vi "总磷氨氮测量数据储存.vi"   [LabVIEW 2016, in "氨氮.lvlib"]
types:
  T1 = cluster{"时间标识":timestamp, "监测值":sgl, "单位":u16, "数据标识":string, "因子编码":u32, "标样参考值":sgl, "F0":sgl, "F1":sgl, "F2":sgl, "F3":sgl, "温度":sgl, "湿度":sgl, "量程标识":string}
  T2 = enum16{"维护数据", "水样测试", "标样核查", "零点核查", "跨度核查", "空白测试", "平行样测试", "加标回收", "空白校准", "标样校准", "初始化（清洗）"}
  T3 = cluster{"系统时间":timestamp, "工作状态":enum16{"空闲", "水样测试", "标样核查", "零点核查", "跨度核查", "空白测试", "平行样测试", "加标回收", "空白校准", "标样校准", "初始化（清洗）"}, "测量模式":enum16{"待机", "连续模式", "周期模式", "定点模式", "受控模式", "手动模式"}, "告警代码":enum16{"无告警", "缺试剂告警", "缺水样告警", "缺蒸馏水告警", "缺标液告警", "仪表漏液告警", "标定异常告警", "超量程告警", "加热异常", "低试剂预警", "超上限告警", "超下限告警", "仪表内部其他异常", "滴定异常告警", "电极异常告警", "量程切换告警", "参数设置告警", "PH电极电位异常", "电导率电极异常", "浊度光度异常", "溶解氧电极异常", "溶解氧光强异常", "温度异常告警", "PH异常告警", "溶解氧异常告警", "电导率异常告警", "浊度异常告警", "叶绿素异常告警", "藻密度异常告警", "蓝绿藻异常告警", "ORP异常告警", "氨氮异常告警", "清洁刷异常告警", "SD卡异常告警", "蓝牙异常告警", "Wifi异常告警", "流程异常告警"}, "故障代码":enum16{"无故障", "电机故障", "温度故障", "通讯故障", "滴定故障"}, "日志代码":u16, "软件版本":u16, "F0":sgl, "F1":sgl, "F2":sgl, "F3":sgl, "T":sgl, "H":sgl, "id":u16, "flowid":u16, "量程":u16, "总磷控温温度1":sgl, "营养盐控温温度2":sgl, "ADC":sgl}
  T4 = enum16{"空闲", "水样测试", "标样核查", "零点核查", "跨度核查", "空白测试", "平行样测试", "加标回收", "空白校准", "标样校准", "初始化（清洗）"}
  T5 = cluster{"跨度值":dbl, "零点标准液浓度":dbl, "跨度标准液浓度":dbl, "标准液标准浓度":dbl}
  T6 = cluster{"因子编码":u32, "单位":u16, "标样参考值":sgl, "水样数据时间":timestamp, "水样实测值":sgl, "水样数据标识":string, "标样数据时间":timestamp, "标样实测值":sgl, "标样数据标识":string, "空白数据时间":timestamp, "空白实测值":sgl, "空白数据标识":string, "零点核查数据时间":timestamp, "零点核查实测值":sgl, "零点核查数据标识":string, "跨度核查数据时间":timestamp, "跨度核查实测值":sgl, "跨度核查数据标识":string, "加标回收数据时间":timestamp, "加标回收实测值":sgl, "加标回收数据标识":string, "平行样数据时间":timestamp, "平行样实测值":sgl, "平行样数据标识":string}
  T7 = cluster{"运行模式":enum16{"维护模式", "常规模式", "应急模式", "质控模式"}}
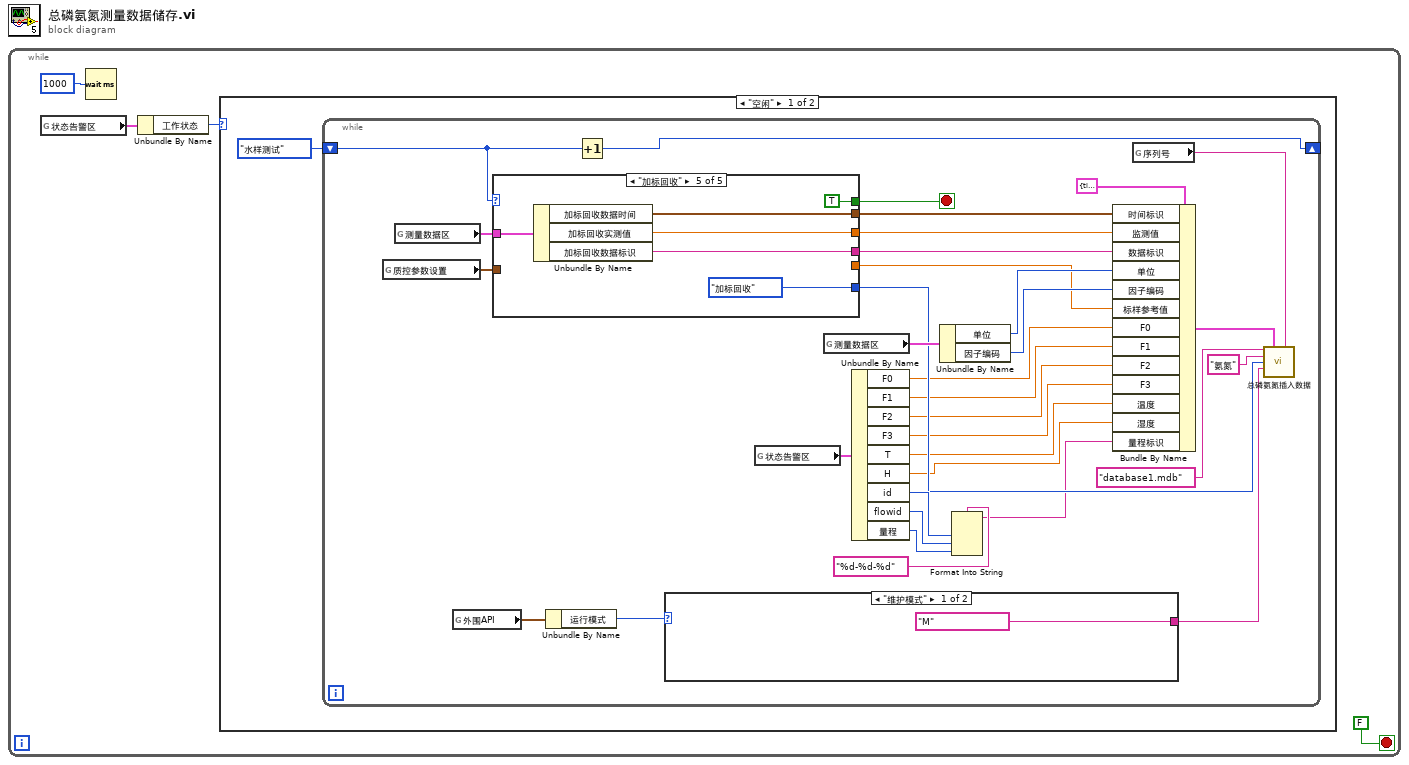
[diagram p0: block diagram]
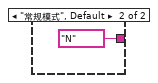
[diagram p2: hidden frame]
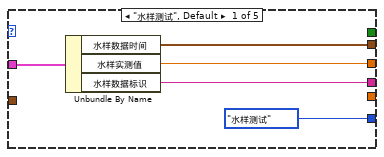
[diagram p3: hidden frame]
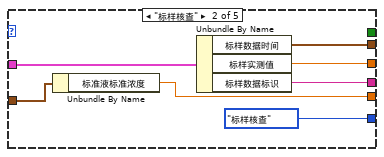
[diagram p4: hidden frame]
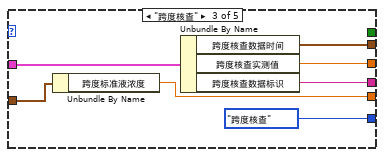
[diagram p5: hidden frame]
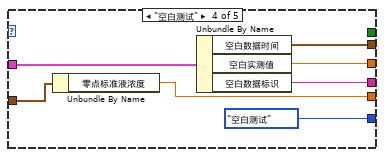
[diagram p6: hidden frame]
diagram:
  n1 = while {
    stop <- FALSE stop-if-true
    n2 = global read "VAR氨氮全局变量.vi" "状态告警区"() -> (w3:T3)
    n3 = Wait (ms)(milliseconds to wait=u32 1000 ("等待时间（毫秒）")) -> ()  [unwired: 1 out]
    n4 = Unbundle By Name(w3) -> ("工作状态"=w2:T4)
    n5 = case shown="\"空闲\"" w2 {
      frame "空闲" {
        n6 = while {
          shift-right: [w32] -> _
          shift-left: enum16{"水样测试", "标样核查", "跨度核查", "空白测试", "加标回收"}."水样测试" ("测量模式") -> [w33]
          stop <- w34 stop-if-true
          n7 = global read "氨氮断电保存全局变量.vi" "质控参数设置"() -> (w7:T5)
          n8 = global read "VAR氨氮全局变量.vi" "测量数据区"() -> (w26:T6)
          n9 = global read "VAR氨氮全局变量.vi" "外围API"() -> (w10:T7)
          n10 = case shown="\"加标回收\"" w33 {
            tunnel: w26 -> [w41 w48 w55 w62 w67]
            tunnel: [w45 w52 w59 w66 w72] -> w31
            tunnel: [w44 w51 w58 w65 w71] -> w30
            tunnel: [w43 w50 w57 w64 w70] -> w29
            tunnel: [T2."水样测试" ("测量模式") T2."标样核查" ("测量模式") T2."跨度核查" ("测量模式") T2."空白测试" ("测量模式") T2."加标回收" ("测量模式")] -> w18
            tunnel: [_ _ _ _ TRUE] -> w34
            tunnel: w7 -> [_ w47 w54 w61 _]
            tunnel: [_ w46 w53 w60 _] -> w6
            frame "水样测试", Default {
              n11 = Unbundle By Name(w41) -> ("水样数据时间"=w45:timestamp, "水样实测值"=w44:sgl, "水样数据标识"=w43:string)
            }
            frame "标样核查" {
              n12 = Unbundle By Name(w47) -> ("标准液标准浓度"=w46:dbl)
              n13 = Unbundle By Name(w48) -> ("标样数据时间"=w52:timestamp, "标样实测值"=w51:sgl, "标样数据标识"=w50:string)
            }
            frame "跨度核查" {
              n14 = Unbundle By Name(w54) -> ("跨度标准液浓度"=w53:dbl)
              n15 = Unbundle By Name(w55) -> ("跨度核查数据时间"=w59:timestamp, "跨度核查实测值"=w58:sgl, "跨度核查数据标识"=w57:string)
            }
            frame "空白测试" {
              n16 = Unbundle By Name(w61) -> ("零点标准液浓度"=w60:dbl)
              n17 = Unbundle By Name(w62) -> ("空白数据时间"=w66:timestamp, "空白实测值"=w65:sgl, "空白数据标识"=w64:string)
            }
            frame "加标回收" {
              n18 = Unbundle By Name(w67) -> ("加标回收数据时间"=w72:timestamp, "加标回收实测值"=w71:sgl, "加标回收数据标识"=w70:string)
            }
          }
          n19 = Unbundle By Name(w10) -> ("运行模式"=w9:enum16{"维护模式", "常规模式", "应急模式", "质控模式"})
          n20 = Increment(x=w33) -> (x+1=w32:enum16{"水样测试", "标样核查", "跨度核查", "空白测试", "加标回收"})
          n21 = case shown="\"维护模式\"" w9 {
            tunnel: ["M" ("数据标记表") "N" ("数据标记表")] -> w8
            frame "维护模式" {
            }
            frame "常规模式", Default {
            }
          }
          n22 = global read "VAR氨氮全局变量.vi" "状态告警区"() -> (w24:T3)
          n23 = global read "VAR氨氮全局变量.vi" "测量数据区"() -> (w25:T6)
          n24 = Unbundle By Name(w24) -> ("F0"=w16:sgl, "F1"=w15:sgl, "F2"=w14:sgl, "F3"=w13:sgl, "T"=w12:sgl, "H"=w11:sgl, "id"=w37:u16, "flowid"=w36:u16, "量程"=w35:u16)
          n25 = Unbundle By Name(w25) -> ("单位"=w28:u16, "因子编码"=w27:u32)
          n26 = Format Into String(format string="%d-%d-%d" ("格式字符串"), w37, w36, w35) -> (resulting string=w17:string)  [unwired: 2 in, 1 out]
          n27 = Bundle By Name(cluster=T1 {"时间标识"=timestamp(0 s since 1904-01-01), "监测值"=0.0, "单位"=0, "数据标识"="", "因子编码"=0, "标样参考值"=0.0, "F0"=0.0, "F1"=0.0, "F2"=0.0, "F3"=0.0, "温度"=0.0, "湿度"=0.0, "量程标识"=""} ("data"), "时间标识"=w31, "监测值"=w30, "数据标识"=w29, "单位"=w28, "因子编码"=w27, "标样参考值"=w6, "F0"=w16, "F1"=w15, "F2"=w14, "F3"=w13, "温度"=w12, "湿度"=w11, "量程标识"=w17) -> (w22:T1)
          n28 = global read "VAR氨氮全局变量.vi" "序列号"() -> (w21:string)
          n29 = call "总磷氨氮插入数据.vi"("database"="database1.mdb", "data"=w22, "SN"=w21, "table"="氨氮", "测量模式"=w18, "数据标记表"=w8) -> ()  [unwired: 9 in, 1 out]
        }
      }
      frame "水样测试", Default {
      }
    }
  }
